vi "Combine xml files_.vi"() -> ()   [LabVIEW 2020]
uses:
  <vilib>/Utility/file.llb/Write Delimited Spreadsheet (string).vi
  XML Handler/XML Handler.lvclass
panel:
  out "Info all":string[][][](array[string])
  in  "XML File Path":path
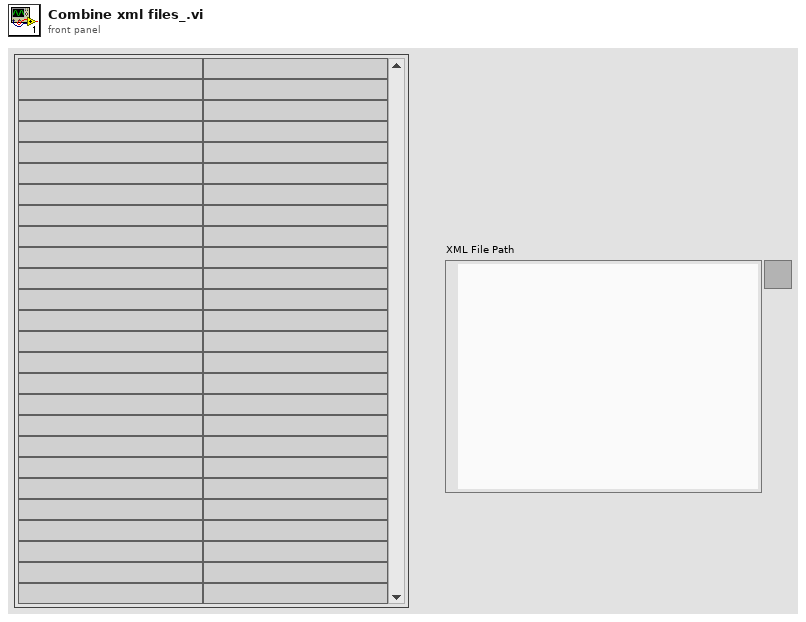
[diagram p1: front panel]
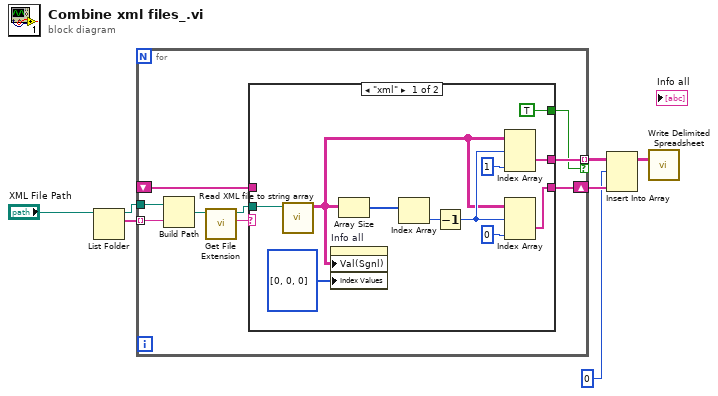
[diagram p0: block diagram]
diagram:
  n1 = List Folder(path="XML File Path") -> (path out=w6:path, filenames=w5:string[])  [unwired: 3 in, 2 out]
  n2 = for {
    tunnel: w6 -> [w16]
    tunnel: w5 -> [w15] mode=indexing
    tunnel: [w12] -> w4 mode=indexing if=w8
    shift-right: [w10] -> w3
    shift-left: _ -> [w9]
    n3 = Build Path(base path=w16, name or relative path=w15) -> (appended path=w14:path)
    n4 = call <vilib>:"Get File Extension.vi"("file"=w14) -> ("lowercase file extension"=w11:string, "dup file"=w13:path)  [unwired: 6 in, 3 out]
    n5 = case shown="\"xml\"" w11 {
      tunnel: w13 -> [w18 _]
      tunnel: [w24 _] -> w12
      tunnel: [w20 w28] -> w10
      tunnel: w9 -> [_ w28]
      tunnel: [TRUE ("replace all? (F)") _] -> w8
      frame "xml" {
        n6 = call "Read XML file to string array.vi"("path to XML document"=w18) -> ("Array"=w17:string[][][])  [unwired: 9 in, 1 out]
        n7 = property on="Info all" class="Arr (strict)"("Val(Sgnl)"=w17, "Index Values"=u32[] [0, 0, 0]) -> ()  [unwired: 2 in, 2 out]
        n8 = Array Size(array=w17) -> (size(s)=w26:i32[])
        n9 = Index Array(array=w26) -> (element=w25:i32)  [unwired: 1 in]
        n10 = Decrement(x=w25) -> (x-1=w21:i32)
        n11 = Index Array(array=w17, index (dim 0)=w21, index (dim 2)=1 ("disabled index (col)")) -> (element=w24:string[])  [unwired: 1 in]
        n12 = Index Array(array=w17, index (dim 0)=w21, index (dim 2)=0 ("disabled index (col)")) -> (element=w20:string[])  [unwired: 1 in]
      }
      frame Default {
      }
    }
  }
  n13 = Insert Into Array(array=w4, index (row)=0, new element=w3) -> (w1:string[][])  [unwired: 1 in]
  n14 = call-poly <vilib>:"Write Delimited Spreadsheet.vi"("2D data"=w1) -> ()  [unwired: 13 in, 2 out]
